vi "Getattribute.vi"(8 "error in (no error)":errorcluster, 11 "OneOfTemplate in":refnum<class "nidaqmx_grpc_GetChanAttributeStringRequest_attribute_enum.lvclass">) -> (0 "error out":errorcluster, 2 "Get_Val":T1, 3 "OneOfTemplate out":refnum<class "nidaqmx_grpc_GetChanAttributeStringRequest_attribute_enum.lvclass">)   [LabVIEW 2021, in "NI_DAQmx_client.lvlib" / "nidaqmx_grpc_GetChanAttributeStringRequest_attribute_enum.lvclass"]
uses:
  nidaqmx_grpc_GetChanAttributeStringRequest_attribute_enum.lvclass
  nidaqmx_grpc_ChannelStringAttribute.ctl
  nidaqmx_grpc_GetChanAttributeStringRequest_attribute_enum.lvclass/nidaqmx_grpc_GetChanAttributeStringRequest_attribute_enum.ctl
  NI_DAQmx_client.lvlib
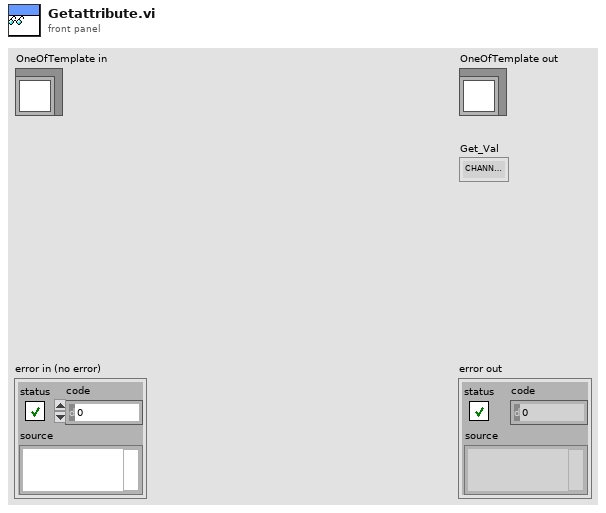
[diagram p1: front panel]
types:
  T1 = typedef "NI_DAQmx_client.lvlib/nidaqmx_grpc_ChannelStringAttribute.ctl" = enum32{"CHANNEL_STRING_ATTRIBUTE_UNSPECIFIED", "CHANNEL_ATTRIBUTE_CI_CTR_TIMEBASE_SRC", "CHANNEL_ATTRIBUTE_CO_CTR_TIMEBASE_SRC", "CHANNEL_ATTRIBUTE_AI_THRMCPL_CJC_CHAN", "CHANNEL_ATTRIBUTE_CI_GPS_SYNC_SRC", "CHANNEL_ATTRIBUTE_AO_CUSTOM_SCALE_NAME", "CHANNEL_ATTRIBUTE_AI_CUSTOM_SCALE_NAME", "CHANNEL_ATTRIBUTE_CI_CUSTOM_SCALE_NAME", "CHANNEL_ATTRIBUTE_CI_FREQ_TERM", "CHANNEL_ATTRIBUTE_CI_PERIOD_TERM", "CHANNEL_ATTRIBUTE_CI_PULSE_WIDTH_TERM", "CHANNEL_ATTRIBUTE_CI_TWO_EDGE_SEP_FIRST_TERM", "CHANNEL_ATTRIBUTE_CI_TWO_EDGE_SEP_SECOND_TERM", "CHANNEL_ATTRIBUTE_CI_SEMI_PERIOD_TERM", "CHANNEL_ATTRIBUTE_CI_COUNT_EDGES_TERM", "CHANNEL_ATTRIBUTE_CO_PULSE_TERM", "CHANNEL_ATTRIBUTE_PHYSICAL_CHAN_NAME", "CHANNEL_ATTRIBUTE_CHAN_DESCR", "CHANNEL_ATTRIBUTE_AI_INPUT_SRC", "CHANNEL_ATTRIBUTE_CI_ENCODER_A_INPUT_TERM", "CHANNEL_ATTRIBUTE_CI_ENCODER_B_INPUT_TERM", "CHANNEL_ATTRIBUTE_CI_ENCODER_Z_INPUT_TERM", "CHANNEL_ATTRIBUTE_AI_TEDS_UNITS", "CHANNEL_ATTRIBUTE_CI_COUNT_EDGES_DIR_TERM", "CHANNEL_ATTRIBUTE_CI_FREQ_DIG_FLTR_TIMEBASE_SRC", "CHANNEL_ATTRIBUTE_CI_PERIOD_DIG_FLTR_TIMEBASE_SRC", "CHANNEL_ATTRIBUTE_CI_COUNT_EDGES_COUNT_DIR_DIG_FLTR_TIMEBASE_SRC", "CHANNEL_ATTRIBUTE_CI_COUNT_EDGES_DIG_FLTR_TIMEBASE_SRC", "CHANNEL_ATTRIBUTE_CI_ENCODER_A_INPUT_DIG_FLTR_TIMEBASE_SRC", "CHANNEL_ATTRIBUTE_CI_ENCODER_B_INPUT_DIG_FLTR_TIMEBASE_SRC", "CHANNEL_ATTRIBUTE_CI_ENCODER_Z_INPUT_DIG_FLTR_TIMEBASE_SRC", "CHANNEL_ATTRIBUTE_CI_PULSE_WIDTH_DIG_FLTR_TIMEBASE_SRC", "CHANNEL_ATTRIBUTE_CI_TWO_EDGE_SEP_FIRST_DIG_FLTR_TIMEBASE_SRC", "CHANNEL_ATTRIBUTE_CI_TWO_EDGE_SEP_SECOND_DIG_FLTR_TIMEBASE_SRC", "CHANNEL_ATTRIBUTE_CI_SEMI_PERIOD_DIG_FLTR_TIMEBASE_SRC", "CHANNEL_ATTRIBUTE_AO_DAC_REF_EXT_SRC", "CHANNEL_ATTRIBUTE_AO_DAC_OFFSET_EXT_SRC", "CHANNEL_ATTRIBUTE_CI_CTR_TIMEBASE_DIG_FLTR_TIMEBASE_SRC", "CHANNEL_ATTRIBUTE_CO_CTR_TIMEBASE_DIG_FLTR_TIMEBASE_SRC", "CHANNEL_ATTRIBUTE_AI_CHAN_CAL_OPERATOR_NAME", "CHANNEL_ATTRIBUTE_AI_CHAN_CAL_DESC", "CHANNEL_ATTRIBUTE_DI_DIG_FLTR_TIMEBASE_SRC", "CHANNEL_ATTRIBUTE_CI_PULSE_FREQ_TERM", "CHANNEL_ATTRIBUTE_CI_PULSE_FREQ_DIG_FLTR_TIMEBASE_SRC", "CHANNEL_ATTRIBUTE_CI_PULSE_TIME_TERM", "CHANNEL_ATTRIBUTE_CI_PULSE_TIME_DIG_FLTR_TIMEBASE_SRC", "CHANNEL_ATTRIBUTE_CI_PULSE_TICKS_TERM", "CHANNEL_ATTRIBUTE_CI_PULSE_TICKS_DIG_FLTR_TIMEBASE_SRC", "CHANNEL_ATTRIBUTE_CI_COUNT_EDGES_COUNT_RESET_TERM", "CHANNEL_ATTRIBUTE_CI_COUNT_EDGES_COUNT_RESET_DIG_FLTR_TIMEBASE_SRC", "CHANNEL_ATTRIBUTE_AI_ROSETTE_STRAIN_GAGE_STRAIN_CHANS", "CHANNEL_ATTRIBUTE_CI_TIMESTAMP_TERM", "CHANNEL_ATTRIBUTE_NAV_CUSTOM_SCALE_NAME", "CHANNEL_ATTRIBUTE_CI_DUTY_CYCLE_TERM", "CHANNEL_ATTRIBUTE_CI_DUTY_CYCLE_DIG_FLTR_TIMEBASE_SRC", "CHANNEL_ATTRIBUTE_CI_VELOCITY_ENCODER_A_INPUT_TERM", "CHANNEL_ATTRIBUTE_CI_VELOCITY_ENCODER_A_INPUT_DIG_FLTR_TIMEBASE_SRC", "CHANNEL_ATTRIBUTE_CI_VELOCITY_ENCODER_B_INPUT_TERM", "CHANNEL_ATTRIBUTE_CI_VELOCITY_ENCODER_B_INPUT_DIG_FLTR_TIMEBASE_SRC", "CHANNEL_ATTRIBUTE_CI_COUNT_EDGES_GATE_TERM", "CHANNEL_ATTRIBUTE_CI_COUNT_EDGES_GATE_DIG_FLTR_TIMEBASE_SRC"}
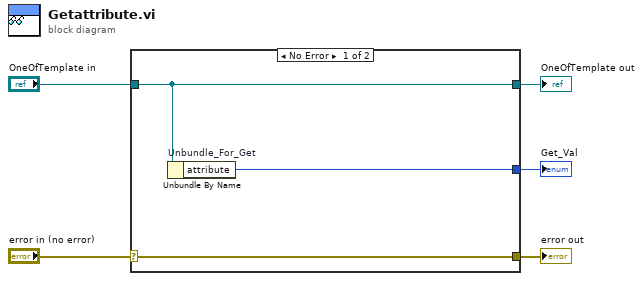
[diagram p0: block diagram]
diagram:
  n1 = case shown="No Error" "error in (no error)" {
    selector: "error in (no error)" -> [w8 w9]
    tunnel: [w8 w9] -> w4
    tunnel: [w7 w10] -> w2
    tunnel: "OneOfTemplate in" -> [w7 w10]
    tunnel: [w6 _] -> w1
    frame No Error {
      n2 = Unbundle By Name "Unbundle_For_Get"(w7) -> ("attribute"=w6:T1)
    }
    frame Error {
    }
  }
  "error out" <- w4
  "OneOfTemplate out" <- w2
  "Get_Val" <- w1
